vi "Quiz04StateMachine.vi"() -> ()   [LabVIEW 2014]
doc: "Use this template to build a user interface event handler design pattern. Use this pattern for dialog boxes and other user interfaces. You also can create and execute user-defined events that the VI can handle the same way as user interface events."
uses:
  Quiz04State.ctl
panel:
  out "Sequence\nRunning":bool
  in  "Run Continuously":bool
  out "Current Test Idx":i32
  in  "Quit":bool
  in  "Interlock":bool
  out "Results":string
  in  "Sequence of tests":u16[](array[ring])=[0, 1, 2] items=["Test 1", "Test 2", "Test 3"]
  in  "Execute Tests":bool
  in  "Stop":bool
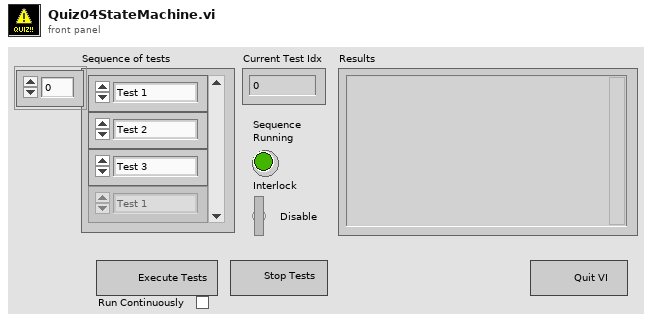
[diagram p1: front panel]
types:
  T1 = typedef "Quiz04State.ctl" = enum16{"Init", "Idle", "CheckError", "Finalize", "StartSequence", "NextTest", "DoTest", "StopSequence"}
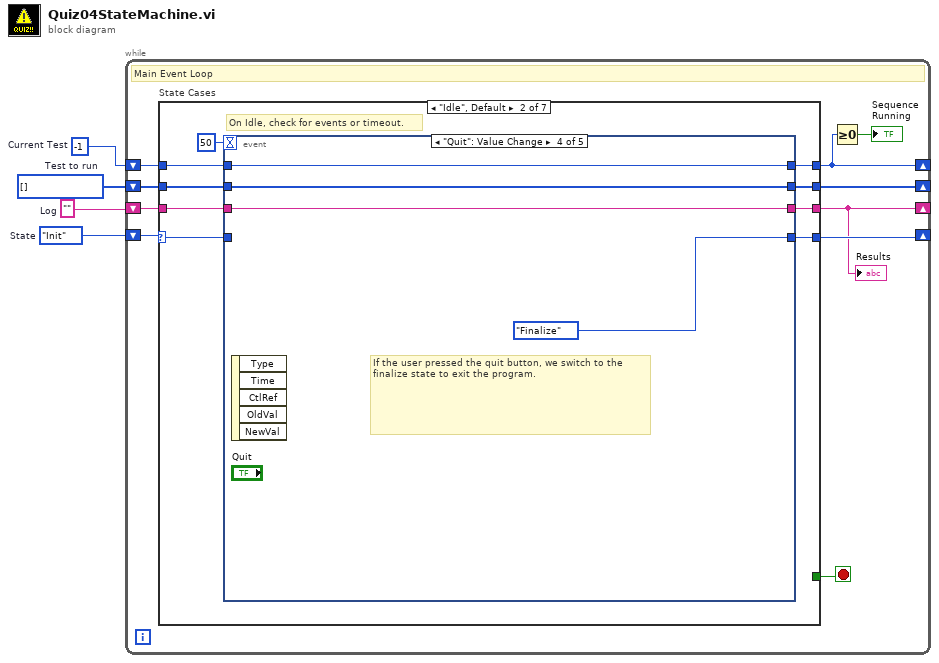
[diagram p0: block diagram]
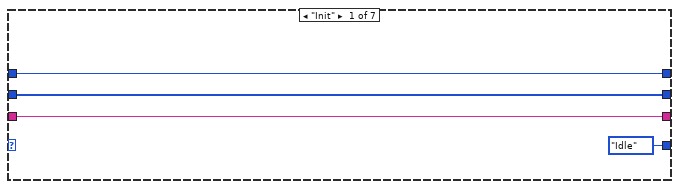
[diagram p2: hidden frame]
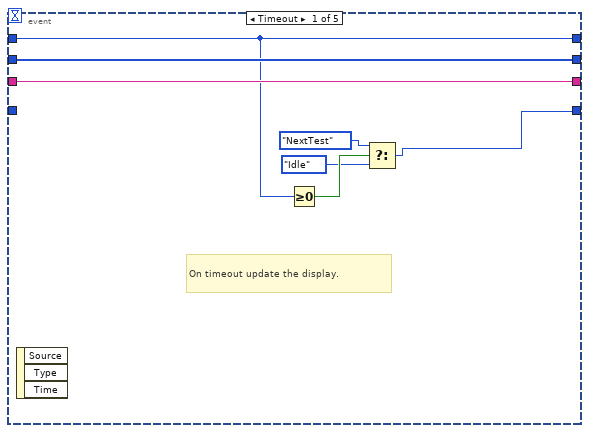
[diagram p3: hidden frame]
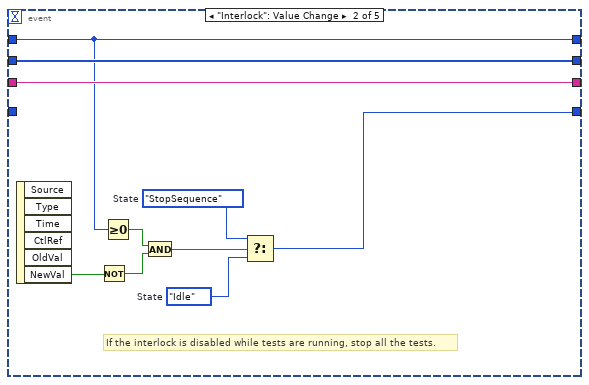
[diagram p4: hidden frame]
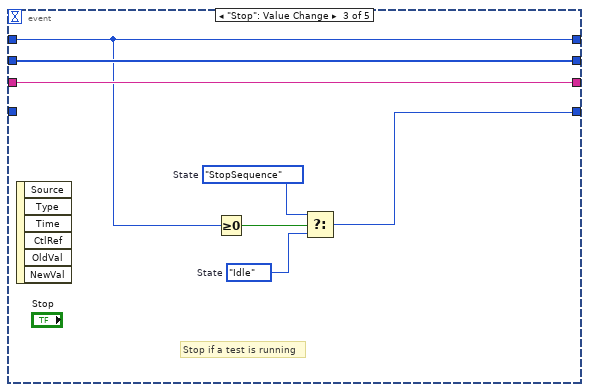
[diagram p5: hidden frame]
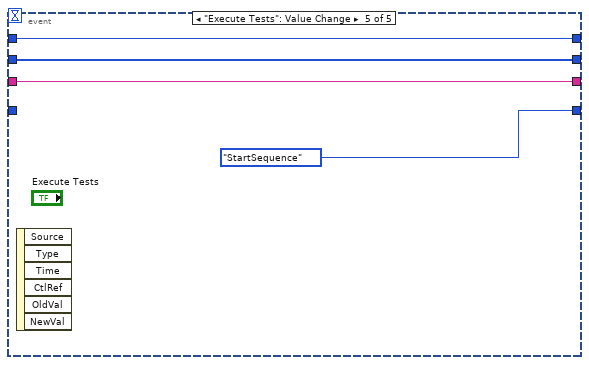
[diagram p6: hidden frame]
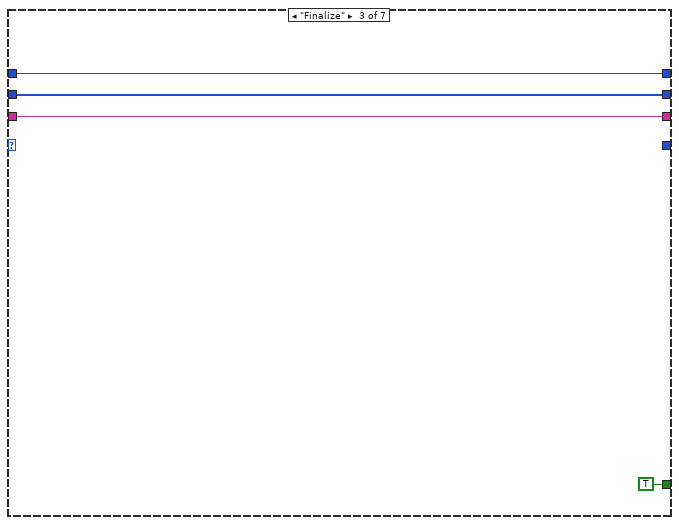
[diagram p7: hidden frame]
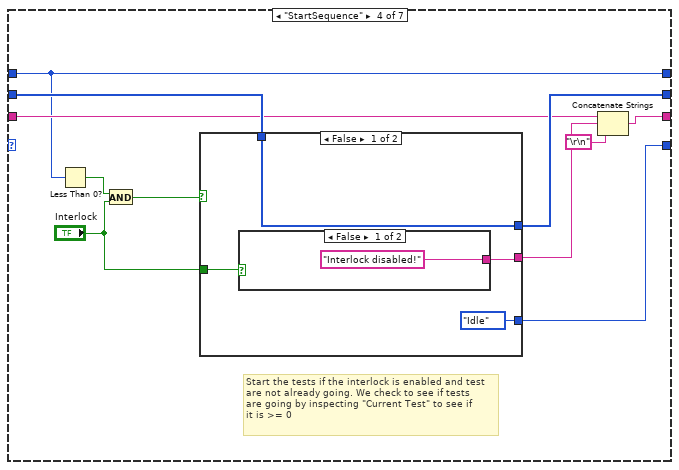
[diagram p8: hidden frame]
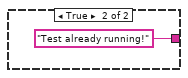
[diagram p9: hidden frame]
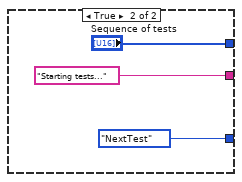
[diagram p10: hidden frame]
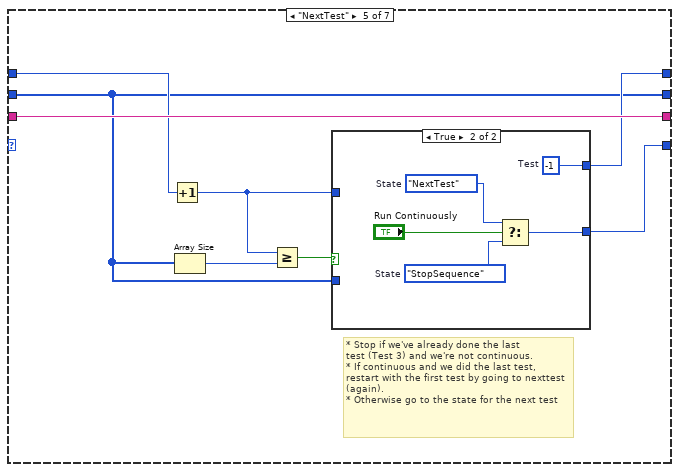
[diagram p11: hidden frame]
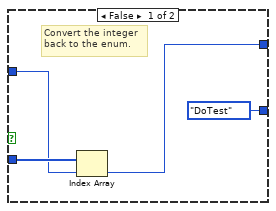
[diagram p12: hidden frame]
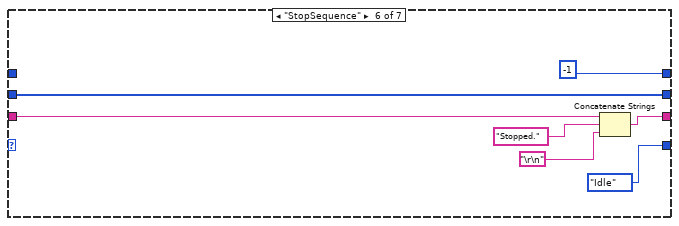
[diagram p13: hidden frame]
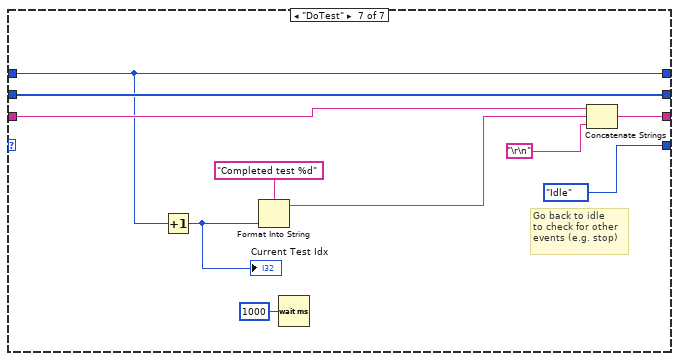
[diagram p14: hidden frame]
diagram:
  w2 = u16[] [] items=["Test 1", "Test 2", "Test 3"]  # Test to run
  w3 = ""  # Log
  w4 = Quiz04State."Init"  # State
  w1 = -1  # Current Test
  n1 = while {
    shift-right: [w5] -> _
    shift-left: w1 -> [w14]
    shift-right: [w12] -> _
    shift-left: w4 -> [w13]
    shift-right: [w11] -> _
    shift-left: w2 -> [w10]
    shift-right: [w7] -> _
    shift-left: w3 -> [w9]
    stop <- w8 stop-if-true
    # "Main Event Loop"
    n2 = case "State Cases" shown="\"Idle\", Default" w13 {
      selector: w13 -> [_ w25 _ _ _ _ _]
      tunnel: w14 -> [w18 w27 w63 w65 w90 _ w112]
      tunnel: [w18 w26 w63 w65 w86 -1 w112] -> w5
      tunnel: [Quiz04State."Idle" ("State") w24 _ w69 w85 Quiz04State."Idle" ("State") Quiz04State."Idle" ("State")] -> w12
      tunnel: [w17 w21 w62 w74 w84 w107 w117] -> w11
      tunnel: w10 -> [w17 w20 w62 w73 w84 w107 w117]
      tunnel: [w16 w23 w61 w66 w91 w101 w114] -> w7
      tunnel: w9 -> [w16 w22 w61 w68 w91 w104 w115]
      tunnel: [_ _ TRUE _ _ _ _] -> w8
      frame "Init" {
      }
      frame "Idle", Default {
        # "On Idle, check for events or timeout."
        # "States"
        n3 = event shown="[3] \"Quit\": Value Change" {
          selector: _ -> [_ _ _ _ _]
          dyn-events: _ -> [_ _ _ _ _]
          timeout: 50 -> [_ _ _ _ _]
          tunnel: w27 -> [w32 w41 w46 w55 w59]
          tunnel: [w32 w41 w46 w55 w59] -> w26
          tunnel: w25 -> [_ _ _ _ _]
          tunnel: [w28 w35 w45 Quiz04State."Finalize" ("State") Quiz04State."StartSequence" ("State")] -> w24
          tunnel: [w33 w43 w50 w53 w57] -> w23
          tunnel: w22 -> [w33 w43 w50 w53 w57]
          tunnel: [w34 w44 w51 w54 w58] -> w21
          tunnel: w20 -> [w34 w44 w51 w54 w58]
          event Timeout {
            # "On timeout update the display."
            n4 = event-data() -> ()  [unwired: 1 in, 3 out]
            n5 = Greater Or Equal To 0?(x=w32) -> (x >= 0?=w31:bool)
            n6 = Select(t=Quiz04State."NextTest" ("State"), s=w31, f=Quiz04State."Idle" ("State")) -> (s? t:f=w28:T1)
          }
          event "Interlock": Value Change {
            w36 = Quiz04State."StopSequence"  # State
            w37 = Quiz04State."Idle"  # State
            # "If the interlock is disabled while tests are running, stop all the tests."
            n7 = event-data() -> ("NewVal"=w42:bool)  [unwired: 1 in, 5 out]
            n8 = Not(x=w42) -> (.not. x?=w39:bool)
            n9 = Greater Or Equal To 0?(x=w41) -> (x >= 0?=w40:bool)
            n10 = And(x=w40, y=w39) -> (x .and. y?=w38:bool)
            n11 = Select(t=w36, s=w38, f=w37) -> (s? t:f=w35:T1)
          }
          event "Stop": Value Change {
            w48 = Quiz04State."StopSequence"  # State
            w49 = Quiz04State."Idle"  # State
            # "Stop if a test is running"
            n12 = event-data() -> ()  [unwired: 1 in, 6 out]
            n13 = Greater Or Equal To 0?(x=w46) -> (x >= 0?=w47:bool)
            n14 = Select(t=w48, s=w47, f=w49) -> (s? t:f=w45:T1)
          }
          event "Quit": Value Change {
            # "If the user pressed the quit button, we switch to the finalize state to exit the program."
            n15 = event-data() -> ()  [unwired: 1 in, 5 out]
          }
          event "Execute Tests": Value Change {
            n16 = event-data() -> ()  [unwired: 1 in, 6 out]
          }
        }
      }
      frame "Finalize" {
      }
      frame "StartSequence" {
        # "Start the tests if the interlock is enabled and test\nare not already going. We check to see if tests\nare going by inspecting \"Current Test\" to see if\nit is >= 0"
        n17 = Less Than 0?(x=w65) -> (x < 0?=w72:bool)
        n18 = And(x=w72, y="Interlock") -> (x .and. y?=w71:bool)
        n19 = case shown="False" w71 {
          tunnel: [w78 "Sequence of tests"] -> w74
          tunnel: w73 -> [w78 _]
          tunnel: "Interlock" -> [w77 _]
          tunnel: [Quiz04State."Idle" ("State") Quiz04State."NextTest" ("State")] -> w69
          tunnel: [w76 "Starting tests..." ("string")] -> w67
          frame False {
            n20 = case shown="False" w77 {
              tunnel: ["Interlock disabled!" ("string") "Test already running!" ("string")] -> w76
              frame False {
              }
              frame True {
              }
            }
          }
          frame True {
          }
        }
        n21 = Concatenate Strings(w68, w67, "\r\n") -> (w66:string)
      }
      frame "NextTest" {
        # "* Stop if we've already done the last\ntest (Test 3) and we're not continuous.\n* If continuous and we did the last test, restart with the first test by going to nexttest (again).\n* Otherwise go to the state for the next test"
        n22 = Increment(x=w90) -> (x+1=w87:i32)
        n23 = Array Size(array=w84) -> (size(s)=w88:i32)
        n24 = Greater Or Equal?(x=w87, y=w88) -> (x >= y?=w89:bool)
        n25 = case shown="True" w89 {
          tunnel: [Quiz04State."DoTest" ("State") w96] -> w85
          tunnel: w87 -> [w94 _]
          tunnel: [w93 w100] -> w86
          tunnel: w84 -> [w95 _]
          frame False {
            # "Convert the integer\nback to the enum."
            n26 = Index Array(array=w95, index=w94) -> (element=w93:u16)
          }
          frame True {
            w97 = Quiz04State."StopSequence"  # State
            w98 = Quiz04State."NextTest"  # State
            w100 = -1  # Test
            n27 = Select(t=w98, s="Run Continuously", f=w97) -> (s? t:f=w96:T1)
          }
        }
      }
      frame "StopSequence" {
        n28 = Concatenate Strings(w104, "Stopped." ("string"), "\r\n") -> (w101:string)
      }
      frame "DoTest" {
        # "Go back to idle\nto check for other\nevents (e.g. stop)"
        n29 = Increment(x=w112) -> (x+1=w109:i32)
        "Current Test Idx" <- w109
        n30 = Format Into String(format string="Completed test %d", w109) -> (resulting string=w111:string)  [unwired: 2 in, 1 out]
        n31 = Wait (ms)(milliseconds to wait=u32 1000) -> ()  [unwired: 1 out]
        n32 = Concatenate Strings(w115, w111, "\r\n") -> (w114:string)
      }
    }
    "Results" <- w7
    n33 = Greater Or Equal To 0?(x=w5) -> (x >= 0?=→"Sequence\nRunning":bool)
  }
